vi "update_crc16.vi"(9 "data":u8, 11 "crc":u16 format="%x") -> (3 "new_crc":u16 format="%.0x")   [LabVIEW 2018]
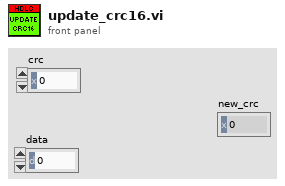
[diagram p1: front panel]
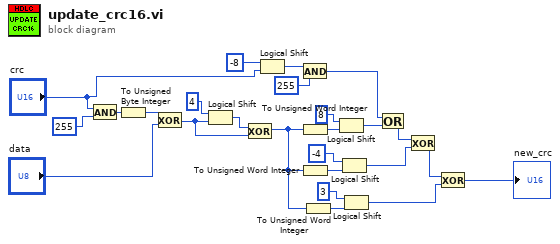
[diagram p0: block diagram]
diagram:
  n1 = And(x="crc", y=u16 255) -> (x .and. y?=w24:u16)
  n2 = To Unsigned Byte Integer(number=w24) -> (unsigned 8bit integer=w23:u8)
  n3 = Exclusive Or(1:"data", 2:w23) -> (0:w19:u8)
  n4 = Logical Shift(y=i16 4, x=w19) -> (x << y=w20:u8)
  n5 = Exclusive Or(1:w19, 2:w20) -> (0:w6:u8)
  n6 = Logical Shift(y=i16 -8, x="crc") -> (x << y=w14:u16)
  n7 = And(x=w14, y=u16 255) -> (x .and. y?=w9:u16)
  n8 = To Unsigned Word Integer(number=w6) -> (unsigned 16bit integer=w10:u16)
  n9 = To Unsigned Word Integer(number=w6) -> (unsigned 16bit integer=w7:u16)
  n10 = To Unsigned Word Integer(number=w6) -> (unsigned 16bit integer=w8:u16)
  n11 = Logical Shift(y=i16 8, x=w10) -> (x << y=w17:u16)
  n12 = Logical Shift(y=i16 -4, x=w7) -> (x << y=w4:u16)
  n13 = Logical Shift(y=i16 3, x=w8) -> (x << y=w2:u16)
  n14 = Or(x=w9, y=w17) -> (x .or. y?=w5:u16)
  n15 = Exclusive Or(1:w4, 2:w5) -> (0:w3:u16)
  n16 = Exclusive Or(1:w2, 2:w3) -> (0:→"new_crc":u16)
